vi "Give Command.vi"(8 "Error In":errorcluster, 9 "Config.ini refnum":T1, 10 "Emotion":string) -> (0 "Error Out":errorcluster, 1 "Boolean_Array":bool[](array[boolean]), 2 "DBL_Array":dbl[](array[numeric]))   [LabVIEW 2017]
doc: "This VI read from the config.ini files and return the boolean & dbl values."
uses:
  <vilib>/Utility/config.llb/Config Data RefNum.ctl
  <vilib>/Utility/config.llb/Read Key (Double).vi
  <vilib>/Utility/config.llb/Read Key (Boolean).vi
  <vilib>/Utility/config.llb/NI_LVConfig.lvlib
panel:
  out "deleted portion":bool
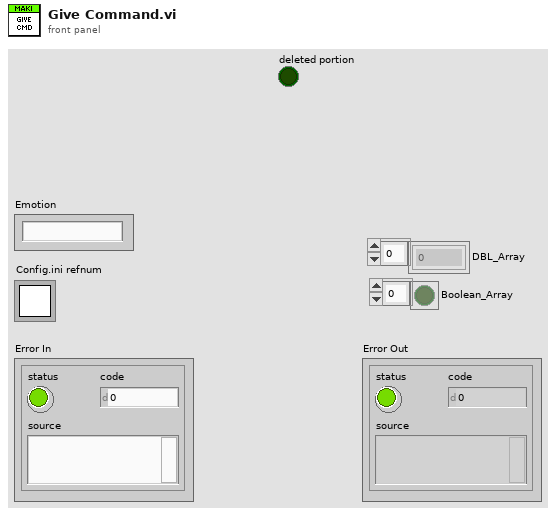
[diagram p1: front panel]
types:
  T1 = typedef "NI_LVConfig.lvlib/Config Data RefNum.ctl" = refnum<k1>
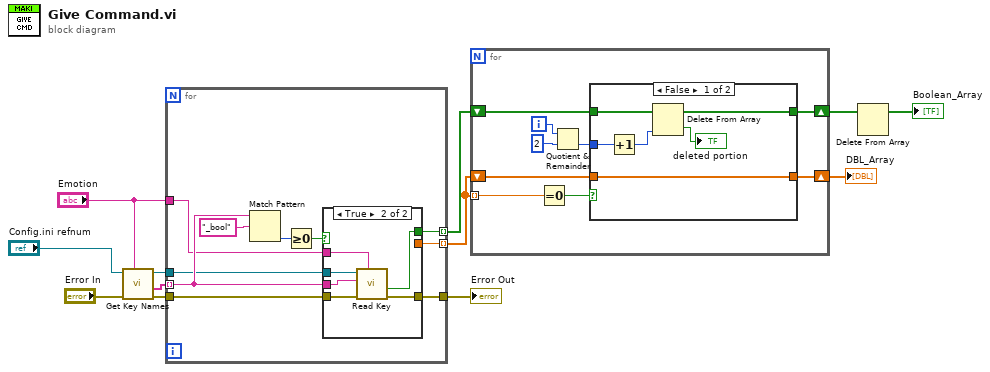
[diagram p0: block diagram]
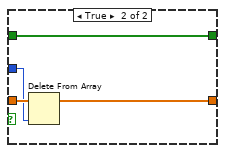
[diagram p2: hidden frame]
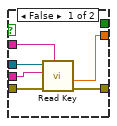
[diagram p3: hidden frame]
diagram:
  n1 = call <vilib>:"Get Key Names.vi"("section"="Emotion", "error in (no error)"="Error In", "refnum"="Config.ini refnum") -> ("error out"=w7:errorcluster, "key names"=w10:string[], "refnum out"=w8:T1)  [unwired: 5 in, 1 out]
  n2 = for {
    tunnel: w10 -> [w19] mode=indexing
    tunnel: "Emotion" -> [w18]
    tunnel: w8 -> [w17]
    tunnel: [w16] -> w5 mode=indexing
    tunnel: [w15] -> w6 mode=indexing
    tunnel: w7 -> [w14]
    tunnel: [w13] -> w1
    n3 = Match Pattern(string=w19, regular expression="_bool") -> (offset past match=w21:i32)  [unwired: 1 in, 3 out]
    n4 = Greater Or Equal To 0?(x=w21) -> (x >= 0?=w20:bool)
    n5 = case shown="True" w20 {
      tunnel: w19 -> [w26 w33]
      tunnel: w18 -> [w27 w34]
      tunnel: w17 -> [w28 w32]
      tunnel: [w25 _] -> w16
      tunnel: [_ w31] -> w15
      tunnel: w14 -> [w24 w30]
      tunnel: [w23 w29] -> w13
      frame False {
        n6 = call-poly <vilib>:"Read Key.vi"("section"=w27, "error in (no error)"=w24, "key"=w26, "refnum"=w28) -> ("error out"=w23:errorcluster, "value"=w25:dbl)  [unwired: 4 in, 2 out]
      }
      frame True {
        n7 = call-poly <vilib>:"Read Key.vi"("section"=w34, "error in (no error)"=w30, "key"=w33, "refnum"=w32) -> ("error out"=w29:errorcluster, "value"=w31:bool)  [unwired: 4 in, 2 out]
      }
    }
  }
  "Error Out" <- w1
  n8 = for {
    tunnel: w5 -> [w43] mode=indexing
    shift-right: [w38] -> w4
    shift-left: w5 -> [w39]
    shift-right: [w36] -> w3
    shift-left: w6 -> [w37]
    i -> [w41]
    n9 = Equal To 0?(x=w43) -> (x = 0?=w42:bool)
    n10 = Quotient & Remainder(x=w41, y=2) -> (floor(x/y)=w35:i32)  [unwired: 1 out]
    n11 = case shown="False" w42 {
      tunnel: w39 -> [w49 w53]
      tunnel: [w49 w52] -> w38
      tunnel: w37 -> [w48 w51]
      tunnel: [w47 w51] -> w36
      tunnel: w35 -> [w46 w50]
      frame False {
        n12 = Increment(x=w46) -> (x+1=w44:i32)
        n13 = Delete From Array(array=w48, index=w44) -> (deleted portion=→"deleted portion":bool, array with subset deleted=w47:bool[])  [unwired: 1 in]
      }
      frame True {
        n14 = Delete From Array(array=w53, index=w50) -> (array with subset deleted=w52:dbl[])  [unwired: 1 in, 1 out]
      }
    }
  }
  "DBL_Array" <- w4
  n15 = Delete From Array(array=w3) -> (array with subset deleted=→"Boolean_Array":bool[])  [unwired: 2 in, 1 out]
